vi "SMTP Email Load Transliteration Tables.vi"(7 "\"Transliterate\" config":string) -> (2 "maps":T1, 3 "charsets":T1)   [LabVIEW 2012, in "NewNI_SMTPEmail.lvlib"]
uses:
  NewNI_SMTPEmail.lvlib
  SMTP Email Keyed Array.ctl
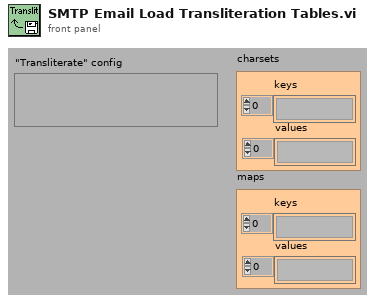
[diagram p1: front panel]
types:
  T1 = typedef "NewNI_SMTPEmail.lvlib/SMTP Email Keyed Array.ctl" = cluster{"keys":string[], "values":string[]}
  T2 = enum16{"read/write", "read-only", "write-only", "write-only (truncate)"}
  T3 = cluster{"token array[0]":string, "token array[1]":string, "token array[2]":string}
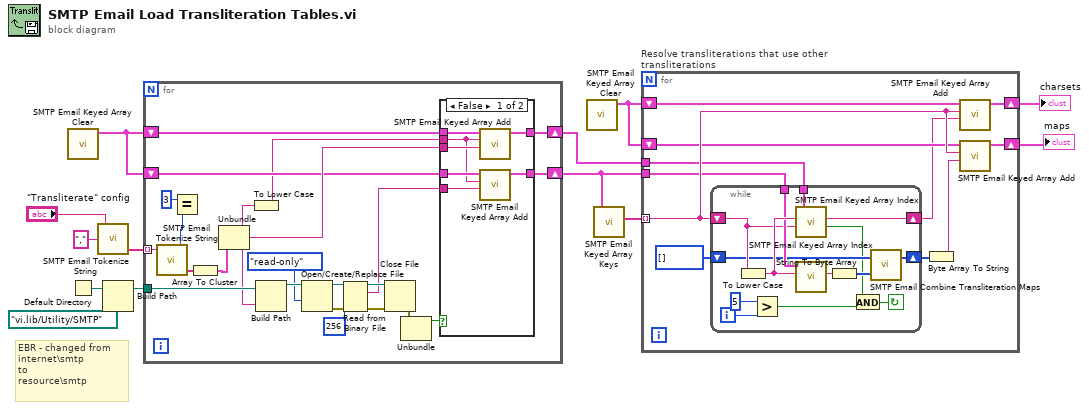
[diagram p0: block diagram]
diagram:
  # "EBR - changed from \ninternet\\smtp\nto\nresource\\smtp"
  n1 = call "SMTP Email Keyed Array Clear.vi"() -> ("array out"=w10:T1)  [unwired: 1 in, 6 out]
  n2 = Default Directory() -> (w3:path)
  n3 = call "SMTP Email Tokenize String.vi"("delimiter ([\\s\\t\\n\\r]+)"="," ("delimiter ([\\s\\t\\n\\r]+)"), "input string"="\"Transliterate\" config") -> ("token array"=w11:string[])  [unwired: 3 out]
  n4 = Build Path(base path=w3, name or relative path=path "vi.lib/Utility/SMTP") -> (appended path=w1:path)
  n5 = for {
    tunnel: w11 -> [w37] mode=indexing
    tunnel: w1 -> [w33]
    shift-right: [w20] -> w4
    shift-left: w10 -> [w21]
    shift-right: [w17] -> w5
    shift-left: w10 -> [w18]
    n6 = call "SMTP Email Tokenize String.vi"("input string"=w37) -> ("token array"=w34:string[], "number of tokens"=w36:i32)  [unwired: 1 in, 2 out]
    n7 = Equal?(x=3, y=w36) -> ()  [unwired: 1 out]
    n8 = Array To Cluster(array=w34) -> (cluster=w22:T3)
    n9 = Unbundle(w22) -> ("token array[0]"=w15:string, "token array[1]"=w19:string, "token array[2]"=w32:string)
    n10 = To Lower Case(string=w15) -> (all lower case string=w14:string)
    n11 = Build Path(base path=w33, name or relative path=w32) -> (appended path=w31:path)
    n12 = Open/Create/Replace File(file path (use dialog)=w31, access (0:read/write)=T2."read-only" ("open mode (0)")) -> (refnum out=w29:refnum<file>, error out=w28:errorcluster)  [unwired: 1 in, 4 out]
    n13 = Read from Binary File(8:w28, 10:256 ("count"), 11:w29) -> (0:w25:errorcluster, 2:w16:string, 3:w26:refnum<file>)  [unwired: 4 out]
    n14 = Close File(refnum=w26, error in=w25) -> (error out=w24:errorcluster)  [unwired: 1 out]
    n15 = Unbundle(w24) -> ("status"=w23:bool)  [unwired: 2 out]
    n16 = case shown="False" w23 {
      tunnel: w21 -> [w44 w46]
      tunnel: [w43 w46] -> w20
      tunnel: w14 -> [w39 _]
      tunnel: w19 -> [w42 _]
      tunnel: w18 -> [w41 w45]
      tunnel: [w40 w45] -> w17
      tunnel: w16 -> [w38 _]
      frame False {
        n17 = call "SMTP Email Keyed Array Add.vi"("value"=w42, "key"=w39, "array in"=w44) -> ("array out"=w43:T1)  [unwired: 1 in, 3 out]
        n18 = call "SMTP Email Keyed Array Add.vi"("value"=w38, "key"=w39, "array in"=w41) -> ("array out"=w40:T1)  [unwired: 1 in, 3 out]
      }
      frame True {
      }
    }
  }
  n19 = call "SMTP Email Keyed Array Clear.vi"() -> ("array out"=w9:T1)  [unwired: 1 in, 6 out]
  n20 = call "SMTP Email Keyed Array Keys.vi"("array in"=w5) -> ("keys"=w6:string[])  [unwired: 6 out]
  n21 = for "Resolve transliterations that use other transliterations" {
    shift-right: [w53] -> w8
    shift-left: w9 -> [w51]
    shift-right: [w52] -> w7
    shift-left: w9 -> [w54]
    tunnel: w6 -> [w55] mode=indexing
    tunnel: w5 -> [w48]
    tunnel: w4 -> [w47]
    n22 = while {
      shift-left: u8[] [] ("map out") -> [w64]
      shift-right: [w63] -> w49
      shift-left: w55 -> [w66]
      shift-right: [w67] -> w50
      tunnel: w47 -> [w68]
      tunnel: w48 -> [w70]
      i -> [w62]
      stop <- w58 continue-if-true
      n23 = To Lower Case(string=w66) -> (all lower case string=w71:string)
      n24 = Greater?(x=5, y=w62) -> (0:w60:bool)
      n25 = call "SMTP Email Keyed Array Index.vi"("default value"=w66, "key"=w71, "array in"=w68) -> ("valid key"=w59:bool, "value"=w67:string)  [unwired: 1 in, 2 out]
      n26 = call "SMTP Email Keyed Array Index.vi"("key"=w71, "array in"=w70) -> ("value"=w69:string)  [unwired: 2 in, 3 out]
      n27 = String To Byte Array(string=w69) -> (unsigned byte array=w65:u8[])
      n28 = And(x=w59, y=w60) -> (x .and. y?=w58:bool)
      n29 = call "SMTP Email Combine Transliteration Maps.vi"("new map"=w65, "map in"=w64) -> ("map out"=w63:u8[])
    }
    n30 = Byte Array To String(unsigned byte array=w49) -> (string=w56:string)
    n31 = call "SMTP Email Keyed Array Add.vi"("value"=w50, "key"=w55, "array in"=w54) -> ("array out"=w52:T1)  [unwired: 1 in, 3 out]
    n32 = call "SMTP Email Keyed Array Add.vi"("value"=w56, "key"=w55, "array in"=w51) -> ("array out"=w53:T1)  [unwired: 1 in, 3 out]
  }
  "charsets" <- w7
  "maps" <- w8
